vi "SV TDMS Write Octave Info.vi"(0 "tdms file":refnum<k34>, 1 "octave info":T6 {"engineering units" items=["custom..."=0, "V"=1, "A"=21, "C"=30, "pC"=31, "s"=32, "-"=29, "Pa"=2, "N"=20, "g"=3, "m/s^2"=4, "m/s"=5, "m"=6, "mm/s"=12, "mm"=13, "micron/s"=14, "micron"=15, "in/s^2"=7, "in/s"=8, "in"=9, "mil/s"=10, "mil"=11, "rad/s^2"=16, "rad/s"=17, "rad"=18, "deg/s^2"=26, "deg/s"=27, "deg"=28, "RPM"=22, "cycle/s^2"=23, "Hz"=24, "cycle"=25, "strain"=19]; "dB reference" format="%.2e"; "weighting filter" items=["Linear", "A-weighting", "B-weighting", "C-weighting", "ITU-R 468-4", "Dolby", "CCITT", "C-message", "Wb", "Wc", "Wd", "We", "Wf", "Wh", "Wj", "Wk", "Wm", "AES17 20 kHz lowpass", "AES17 40 kHz lowpass", "AES17 20 kHz highpass", "AES17 40 kHz highpass"]}, 5 "group name in":string, 7 "channel name in":string, 11 "error in":errorcluster) -> (4 "tdms file out":refnum<k34>, 6 "group name out":string, 8 "channel name out":string, 13 "function info":T5 {"function type" items=["Signal"=0, "Speed"=3, "Ratio"=6, "Count"=7, "-"=9, "Level"=10, "-"=19, "Octave Spectrum"=20, "-"=29, "FFT Auto Spectrum"=30, "FFT Cross Spectrum"=40, "Frequency Response"=50, "-"=59, "Event"=90]; "function subtype" items=["Unscaled binary"=0, "Scaled voltage"=1, "Scaled engineering units"=2, "-"=10, "Value"=19, "DC"=11, "AC"=12, "RMS^2"=13, "RMS"=14, "Peak"=15, "Peak to peak"=16, "-"=20, "1/1 octave"=21, "1/3 octave"=22, "1/6 octave"=23, "1/12 octave"=24, "1/24 octave"=25, "-"=30, "Density"=31, "Magnitude"=32, "Phase"=33, "Real"=34, "Imaginary"=35, "Complex"=345, "Coherence"=36, "-"=90, "Unknown"=99]; "X-domain" items=["Time (s)"=0, "Frequency-CB (Hz)"=1, "Frequency-CPB (Hz)"=1248, "Frequency-Arbitrary (Hz)"=2357, "Quefrency (s)"=2, "Revolutions (rev)"=3, "Order"=4, "Speed (RPM)"=11, "Speed (rad/s)"=21, "Index"=65535]}, 14 "unit info":T1, 15 "error out":errorcluster)   [LabVIEW 2017]
uses:
  <vilib>/addons/_NISVFA/_Shared subVIs/Controls/svc_Octave Info.ctl
  <vilib>/addons/_NISVFA/_Shared subVIs/Controls/svc_Octave Standard.ctl
  <vilib>/addons/_NISVFA/_Shared subVIs/Controls/svc_Weighting Filter Text Ring.ctl
  <vilib>/addons/_NISVFA/_Shared subVIs/Controls/svc_Engineering Units Text Ring.ctl
  <vilib>/addons/_NISVFA/_Shared subVIs/Controls/NI Function Type.ctl
  <vilib>/addons/_NISVFA/_Shared subVIs/Controls/NI Function SubType.ctl
  <vilib>/addons/_NISVFA/_Shared subVIs/Controls/svc_X-Axis Units.ctl
  <vilib>/addons/_NISVFA/_Shared subVIs/Controls/NI Channel Properties.ctl
  <vilib>/addons/_NISVFA/_Shared subVIs/Controls/SV Channel Properties.ctl
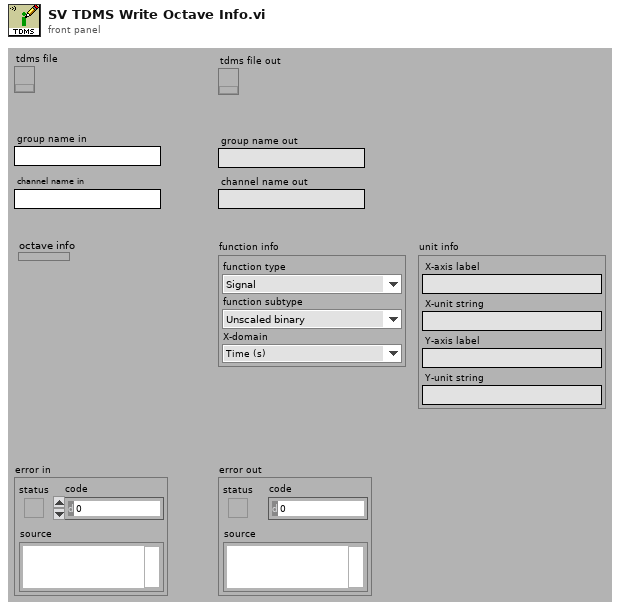
[diagram p1: front panel]
types:
  T1 = cluster{"X-axis label":string, "X-unit string":string, "Y-axis label":string, "Y-unit string":string}
  T2 = typedef "NI Function Type.ctl" = u16
  T3 = typedef "NI Function SubType.ctl" = u16
  T4 = typedef "svc_X-Axis Units.ctl" = u16
  T5 = cluster{"function type":T2, "function subtype":T3, "X-domain":T4}
  T6 = typedef "svc_Octave Info.ctl" = cluster{"standard":T7, "bandwidth":enum16{"1 octave", "1/3 octave", "1/6 octave", "1/12 octave", "1/24 octave"}, "low band":i32, "high band":i32, "weighting filter":T8, "dB reference":dbl, "dB On":bool, "unit label":string, "channel name":string, "description":string, "engineering units":T9, "custom label":string, "spectrum type":enum16{"power", "magnitude"}, "spectral density":bool, "filters settled":bool}
  T7 = typedef "svc_Octave Standard.ctl" = enum16{"ANSI S1.11", "IEC 61260"}
  T8 = typedef "svc_Weighting Filter Text Ring.ctl" = u16
  T9 = typedef "svc_Engineering Units Text Ring.ctl" = u16
  T10 = typedef "NI Channel Properties.ctl" = u16
  T11 = typedef "SV Channel Properties.ctl" = u16
  T12 = enum16{"1 octave", "1/3 octave", "1/6 octave", "1/12 octave", "1/24 octave"}
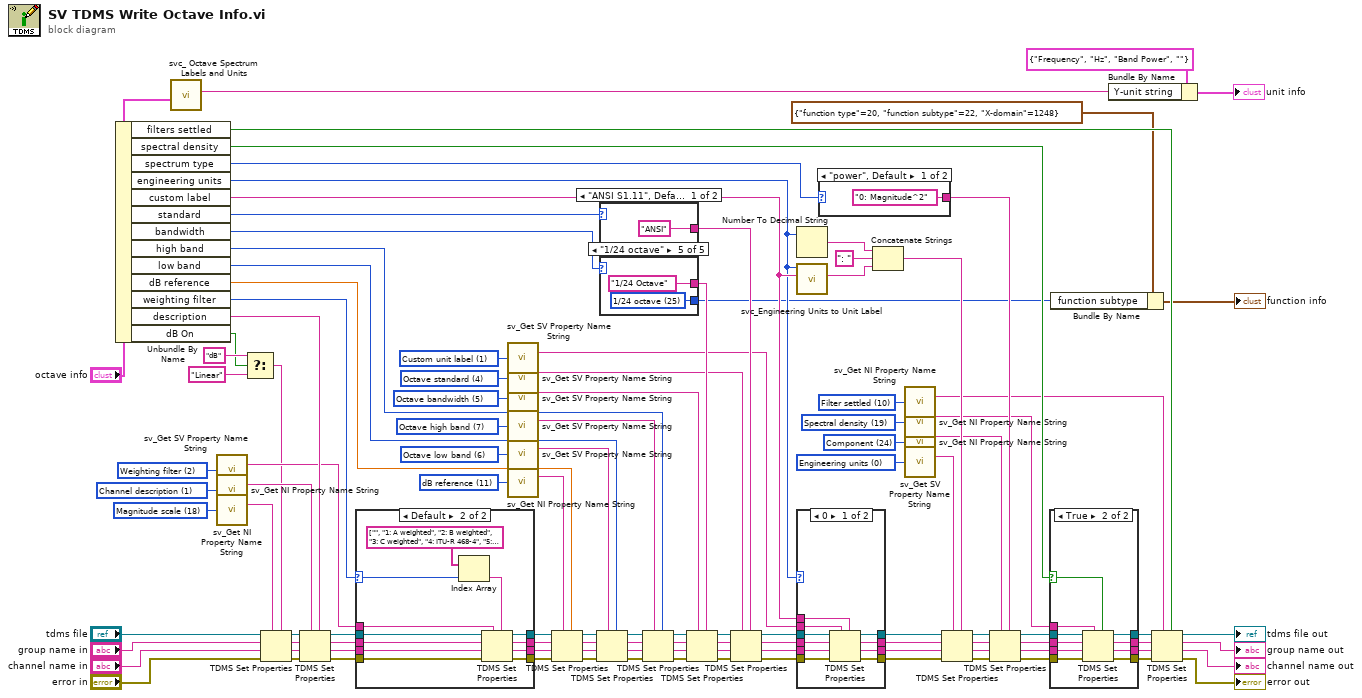
[diagram p0: block diagram]
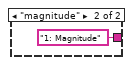
[diagram p2: hidden frame]
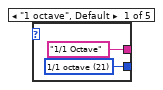
[diagram p6: hidden frame]
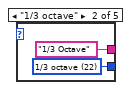
[diagram p7: hidden frame]
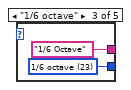
[diagram p8: hidden frame]
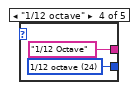
[diagram p9: hidden frame]
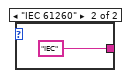
[diagram p10: hidden frame]
diagram:
  w29 = T10 24 items=["Channel name", "Channel description", "Y-axis label", "Y-axis unit string", "X-axis label", "X-axis unit string", "x0", "dx", "Number of samples", "X channel", "Filter settled", "dB reference", "Window", "Window parameter", "Window size", "FFT size", "Peak units", "Spectrum type", "Magnitude scale", "Spectral density", "Sensor sensitivity (mV/EU)", "X-axis domain", "LabVIEW datatype", "Function type", "Component", "Level detector"] ("property")
  w49 = T11 1 items=["Engineering units", "Custom unit label", "Weighting filter", "Pregain", "Octave standard", "Octave bandwidth", "Octave low band", "Octave high band", "Spectrum skewed"] ("SV property")
  w39 = T11 4 items=["Engineering units", "Custom unit label", "Weighting filter", "Pregain", "Octave standard", "Octave bandwidth", "Octave low band", "Octave high band", "Spectrum skewed"] ("SV property")
  w40 = T11 5 items=["Engineering units", "Custom unit label", "Weighting filter", "Pregain", "Octave standard", "Octave bandwidth", "Octave low band", "Octave high band", "Spectrum skewed"] ("SV property")
  w47 = T11 7 items=["Engineering units", "Custom unit label", "Weighting filter", "Pregain", "Octave standard", "Octave bandwidth", "Octave low band", "Octave high band", "Spectrum skewed"] ("SV property")
  w48 = T11 6 items=["Engineering units", "Custom unit label", "Weighting filter", "Pregain", "Octave standard", "Octave bandwidth", "Octave low band", "Octave high band", "Spectrum skewed"] ("SV property")
  w51 = T11 0 items=["Engineering units", "Custom unit label", "Weighting filter", "Pregain", "Octave standard", "Octave bandwidth", "Octave low band", "Octave high band", "Spectrum skewed"] ("SV property")
  w41 = T11 2 items=["Engineering units", "Custom unit label", "Weighting filter", "Pregain", "Octave standard", "Octave bandwidth", "Octave low band", "Octave high band", "Spectrum skewed"] ("SV property")
  w44 = T10 11 items=["Channel name", "Channel description", "Y-axis label", "Y-axis unit string", "X-axis label", "X-axis unit string", "x0", "dx", "Number of samples", "X channel", "Filter settled", "dB reference", "Window", "Window parameter", "Window size", "FFT size", "Peak units", "Spectrum type", "Magnitude scale", "Spectral density"] ("property")
  w45 = T10 1 items=["Channel name", "Channel description", "Y-axis label", "Y-axis unit string", "X-axis label", "X-axis unit string", "x0", "dx", "Number of samples", "X channel", "Filter settled", "dB reference", "Window", "Window parameter", "Window size", "FFT size", "Peak units", "Spectrum type", "Magnitude scale", "Spectral density"] ("property")
  w46 = T10 18 items=["Channel name", "Channel description", "Y-axis label", "Y-axis unit string", "X-axis label", "X-axis unit string", "x0", "dx", "Number of samples", "X channel", "Filter settled", "dB reference", "Window", "Window parameter", "Window size", "FFT size", "Peak units", "Spectrum type", "Magnitude scale", "Spectral density"] ("property")
  w50 = T10 19 items=["Channel name", "Channel description", "Y-axis label", "Y-axis unit string", "X-axis label", "X-axis unit string", "x0", "dx", "Number of samples", "X channel", "Filter settled", "dB reference", "Window", "Window parameter", "Window size", "FFT size", "Peak units", "Spectrum type", "Magnitude scale", "Spectral density"] ("property")
  w52 = T10 10 items=["Channel name", "Channel description", "Y-axis label", "Y-axis unit string", "X-axis label", "X-axis unit string", "x0", "dx", "Number of samples", "X channel", "Filter settled", "dB reference", "Window", "Window parameter", "Window size", "FFT size", "Peak units", "Spectrum type", "Magnitude scale", "Spectral density"] ("property")
  n1 = Unbundle By Name("octave info") -> ("filters settled"=w108:bool, "spectral density"=w100:bool, "spectrum type"=w54:enum16{"power", "magnitude"}, "engineering units"=w61:T9, "custom label"=w62:string, "standard"=w95:T7, "bandwidth"=w97:T12, "high band"=w1:i32, "low band"=w2:i32, "dB reference"=w3:dbl, "weighting filter"=w59:T8, "description"=w84:string, "dB On"=w18:bool)
  n2 = call <vilib>:"svc_ Octave Spectrum Labels and Units.vi"("octave info"="octave info") -> ("unit label"=w20:string)  [unwired: 9 in, 1 out]
  n3 = call <vilib>:"sv_Get SV Property Name String.vi"("property"=w41) -> ("TDMS property name"=w37:string)  [unwired: 13 in, 1 out]
  n4 = call <vilib>:"sv_Get NI Property Name String.vi"("property"=w45) -> ("TDMS property name"=w38:string)  [unwired: 13 in, 1 out]
  n5 = call <vilib>:"sv_Get NI Property Name String.vi"("property"=w46) -> ("TDMS property name"=w16:string)  [unwired: 13 in, 1 out]
  n6 = Select(t="dB" ("f"), s=w18, f="Linear" ("t")) -> (s? t:f=w17:string)
  n7 = TDMS Set Properties(5:w17, 7:w16, 8:"error in", 9:"channel name in", 10:"group name in", 11:"tdms file") -> (0:w85:errorcluster, 1:w88:string, 2:w87:string, 3:w86:refnum<k34>)
  n8 = TDMS Set Properties(5:w84, 7:w38, 8:w85, 9:w88, 10:w87, 11:w86) -> (0:w8:errorcluster, 1:w9:string, 2:w10:string, 3:w11:refnum<k34>)
  n9 = case shown="Default" w59 {
    selector: w59 -> [_ w119]
    tunnel: w8 -> [w113 w128]
    tunnel: w9 -> [w114 w127]
    tunnel: w10 -> [w115 w126]
    tunnel: w11 -> [w116 w125]
    tunnel: [w116 w124] -> w58
    tunnel: [w115 w123] -> w57
    tunnel: [w114 w122] -> w56
    tunnel: [w113 w121] -> w55
    tunnel: w37 -> [_ w120]
    frame 0 {
    }
    frame Default {
      n10 = Index Array(array=string[] ["", "1: A weighted", "2: B weighted", "3: C weighted", "4: ITU-R 468-4", "5: Dolby", "6: CCITT", "7: C-message", "8: Wb", "9: Wc", "10: Wd", "11: We", "12: Wf", "13: Wh", "14: Wj", "15: Wk", "16: Wm"] ("transposed array"), index=w119) -> (element=w118:string)
      n11 = TDMS Set Properties(5:w118, 7:w120, 8:w128, 9:w127, 10:w126, 11:w125) -> (0:w121:errorcluster, 1:w122:string, 2:w123:string, 3:w124:refnum<k34>)
    }
  }
  n12 = call <vilib>:"sv_Get SV Property Name String.vi"("property"=w49) -> ("TDMS property name"=w31:string)  [unwired: 13 in, 1 out]
  n13 = call <vilib>:"sv_Get SV Property Name String.vi"("property"=w39) -> ("TDMS property name"=w32:string)  [unwired: 13 in, 1 out]
  n14 = call <vilib>:"sv_Get SV Property Name String.vi"("property"=w40) -> ("TDMS property name"=w33:string)  [unwired: 13 in, 1 out]
  n15 = call <vilib>:"sv_Get SV Property Name String.vi"("property"=w47) -> ("TDMS property name"=w34:string)  [unwired: 13 in, 1 out]
  n16 = call <vilib>:"sv_Get SV Property Name String.vi"("property"=w48) -> ("TDMS property name"=w35:string)  [unwired: 13 in, 1 out]
  n17 = call <vilib>:"sv_Get NI Property Name String.vi"("property"=w44) -> ("TDMS property name"=w36:string)  [unwired: 13 in, 1 out]
  n18 = TDMS Set Properties(5:w3, 7:w36, 8:w55, 9:w56, 10:w57, 11:w58) -> (0:w76:errorcluster, 1:w77:string, 2:w78:string, 3:w79:refnum<k34>)
  n19 = TDMS Set Properties(5:w2, 7:w35, 8:w76, 9:w77, 10:w78, 11:w79) -> (0:w92:errorcluster, 1:w91:string, 2:w90:string, 3:w89:refnum<k34>)
  n20 = case shown="\"ANSI S1.11\", Default" w95 {
    tunnel: ["ANSI" ("f") "IEC" ("f")] -> w96
    frame "ANSI S1.11", Default {
    }
    frame "IEC 61260" {
    }
  }
  n21 = case shown="\"1/24 octave\"" w97 {
    tunnel: ["1/1 Octave" ("f") "1/3 Octave" ("f") "1/6 Octave" ("f") "1/12 Octave" ("f") "1/24 Octave" ("f")] -> w98
    tunnel: [w131 w133 w135 w137 w139] -> w22
    frame "1 octave", Default {
      w131 = T3 21 items=["Unscaled binary"=0, "Scaled voltage"=1, "Scaled engineering units"=2, "-"=10, "Value"=19, "DC"=11, "AC"=12, "RMS^2"=13, "RMS"=14, "Peak"=15, "Peak to peak"=16, "-"=20, "1/1 octave"=21, "1/3 octave"=22, "1/6 octave"=23, "1/12 octave"=24, "1/24 octave"=25, "-"=30, "Density"=31, "Magnitude"=32, "Phase"=33, "Real"=34, "Imaginary"=35, "Complex"=345, "Coherence"=36, "-"=90, "Unknown"=99] ("function subtype")
    }
    frame "1/3 octave" {
      w133 = T3 22 items=["Unscaled binary"=0, "Scaled voltage"=1, "Scaled engineering units"=2, "-"=10, "Value"=19, "DC"=11, "AC"=12, "RMS^2"=13, "RMS"=14, "Peak"=15, "Peak to peak"=16, "-"=20, "1/1 octave"=21, "1/3 octave"=22, "1/6 octave"=23, "1/12 octave"=24, "1/24 octave"=25, "-"=30, "Density"=31, "Magnitude"=32, "Phase"=33, "Real"=34, "Imaginary"=35, "Complex"=345, "Coherence"=36, "-"=90, "Unknown"=99] ("function subtype")
    }
    frame "1/6 octave" {
      w135 = T3 23 items=["Unscaled binary"=0, "Scaled voltage"=1, "Scaled engineering units"=2, "-"=10, "Value"=19, "DC"=11, "AC"=12, "RMS^2"=13, "RMS"=14, "Peak"=15, "Peak to peak"=16, "-"=20, "1/1 octave"=21, "1/3 octave"=22, "1/6 octave"=23, "1/12 octave"=24, "1/24 octave"=25, "-"=30, "Density"=31, "Magnitude"=32, "Phase"=33, "Real"=34, "Imaginary"=35, "Complex"=345, "Coherence"=36, "-"=90, "Unknown"=99] ("function subtype")
    }
    frame "1/12 octave" {
      w137 = T3 24 items=["Unscaled binary"=0, "Scaled voltage"=1, "Scaled engineering units"=2, "-"=10, "Value"=19, "DC"=11, "AC"=12, "RMS^2"=13, "RMS"=14, "Peak"=15, "Peak to peak"=16, "-"=20, "1/1 octave"=21, "1/3 octave"=22, "1/6 octave"=23, "1/12 octave"=24, "1/24 octave"=25, "-"=30, "Density"=31, "Magnitude"=32, "Phase"=33, "Real"=34, "Imaginary"=35, "Complex"=345, "Coherence"=36, "-"=90, "Unknown"=99] ("function subtype")
    }
    frame "1/24 octave" {
      w139 = T3 25 items=["Unscaled binary"=0, "Scaled voltage"=1, "Scaled engineering units"=2, "-"=10, "Value"=19, "DC"=11, "AC"=12, "RMS^2"=13, "RMS"=14, "Peak"=15, "Peak to peak"=16, "-"=20, "1/1 octave"=21, "1/3 octave"=22, "1/6 octave"=23, "1/12 octave"=24, "1/24 octave"=25, "-"=30, "Density"=31, "Magnitude"=32, "Phase"=33, "Real"=34, "Imaginary"=35, "Complex"=345, "Coherence"=36, "-"=90, "Unknown"=99] ("function subtype")
    }
  }
  n22 = TDMS Set Properties(5:w1, 7:w34, 8:w92, 9:w91, 10:w90, 11:w89) -> (0:w12:errorcluster, 1:w13:string, 2:w14:string, 3:w15:refnum<k34>)
  n23 = TDMS Set Properties(5:w98, 7:w33, 8:w12, 9:w13, 10:w14, 11:w15) -> (0:w83:errorcluster, 1:w82:string, 2:w81:string, 3:w80:refnum<k34>)
  n24 = TDMS Set Properties(5:w96, 7:w32, 8:w83, 9:w82, 10:w81, 11:w80) -> (0:w72:errorcluster, 1:w73:string, 2:w74:string, 3:w75:refnum<k34>)
  n25 = Number To Decimal String(number=w61) -> (decimal integer string=w27:string)  [unwired: 1 in]
  n26 = call <vilib>:"svc_Engineering Units to Unit Label.vi"("custom label"=w62, "engineering units"=w61) -> ("unit label"=w26:string)  [unwired: 8 in, 1 out]
  n27 = case shown="0" w61 {
    tunnel: w72 -> [w150 w151]
    tunnel: w73 -> [w149 w152]
    tunnel: w74 -> [w148 w153]
    tunnel: w75 -> [w147 w154]
    tunnel: [w146 w154] -> w71
    tunnel: [w145 w153] -> w70
    tunnel: [w144 w152] -> w69
    tunnel: [w143 w151] -> w68
    tunnel: w31 -> [w142 _]
    tunnel: w62 -> [w141 _]
    frame 0 {
      n28 = TDMS Set Properties(5:w141, 7:w142, 8:w150, 9:w149, 10:w148, 11:w147) -> (0:w143:errorcluster, 1:w144:string, 2:w145:string, 3:w146:refnum<k34>)
    }
    frame Default {
    }
  }
  n29 = case shown="\"power\", Default" w54 {
    tunnel: ["0: Magnitude^2" ("f") "1: Magnitude" ("f")] -> w53
    frame "power", Default {
    }
    frame "magnitude" {
    }
  }
  n30 = Concatenate Strings(w27, ": " ("string"), w26) -> (w60:string)
  n31 = call <vilib>:"sv_Get NI Property Name String.vi"("property"=w52) -> ("TDMS property name"=w43:string)  [unwired: 13 in, 1 out]
  n32 = call <vilib>:"sv_Get NI Property Name String.vi"("property"=w50) -> ("TDMS property name"=w42:string)  [unwired: 13 in, 1 out]
  n33 = call <vilib>:"sv_Get NI Property Name String.vi"("property"=w29) -> ("TDMS property name"=w28:string)  [unwired: 13 in, 1 out]
  n34 = call <vilib>:"sv_Get SV Property Name String.vi"("property"=w51) -> ("TDMS property name"=w30:string)  [unwired: 13 in, 1 out]
  n35 = TDMS Set Properties(5:w60, 7:w30, 8:w68, 9:w69, 10:w70, 11:w71) -> (0:w64:errorcluster, 1:w65:string, 2:w66:string, 3:w67:refnum<k34>)
  n36 = TDMS Set Properties(5:w53, 7:w28, 8:w64, 9:w65, 10:w66, 11:w67) -> (0:w103:errorcluster, 1:w102:string, 2:w101:string, 3:w99:refnum<k34>)
  n37 = case shown="True" w100 {
    selector: w100 -> [_ w162]
    tunnel: w103 -> [w157 w170]
    tunnel: w102 -> [w158 w169]
    tunnel: w101 -> [w159 w168]
    tunnel: w99 -> [w160 w167]
    tunnel: [w160 w166] -> w107
    tunnel: [w159 w165] -> w106
    tunnel: [w158 w164] -> w105
    tunnel: [w157 w163] -> w104
    tunnel: w42 -> [_ w161]
    frame False {
    }
    frame True {
      n38 = TDMS Set Properties(5:w162, 7:w161, 8:w170, 9:w169, 10:w168, 11:w167) -> (0:w163:errorcluster, 1:w164:string, 2:w165:string, 3:w166:refnum<k34>)
    }
  }
  n39 = Bundle By Name(cluster=T5 {"function type"=20, "function subtype"=22, "X-domain"=1248} ("function info"), "function subtype"=w22) -> (→"function info":T5)
  n40 = Bundle By Name(cluster=T1 {"X-axis label"="Frequency", "X-unit string"="Hz", "Y-axis label"="Band Power", "Y-unit string"=""} ("unit info"), "Y-unit string"=w20) -> (→"unit info":T1)
  n41 = TDMS Set Properties(5:w108, 7:w43, 8:w104, 9:w105, 10:w106, 11:w107) -> (0:→"error out":errorcluster, 1:→"channel name out":string, 2:→"group name out":string, 3:→"tdms file out":refnum<k34>)
